vi "IIC Write Bytes.vi"(5 "TimeOutMs":i32, 6 "WriteLen":i32, 7 "pWriteData":u8[](array[numeric])=array[4097 elements], 9 "SlaveAddr":i16, 10 "IICIndex":i32, 11 "DevHandle":i32) -> (2 "function return":i32, 3 "pWriteData out":u8[](array[numeric]))   [LabVIEW 2010, in "usb2iic.lvlib"]
doc: "int WINAPI IIC_WriteBytes(int DevHandle,int IICIndex,short SlaveAddr,unsigned char *pWriteData,int WriteLen,int TimeOutMs);"
uses:
  usb2iic.lvlib
  USB2XXX.dll
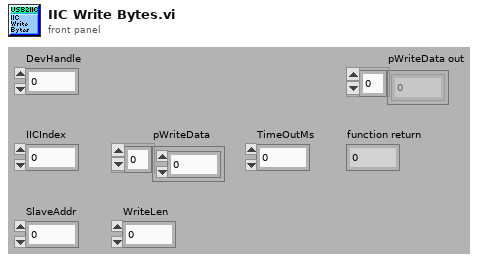
[diagram p1: front panel]
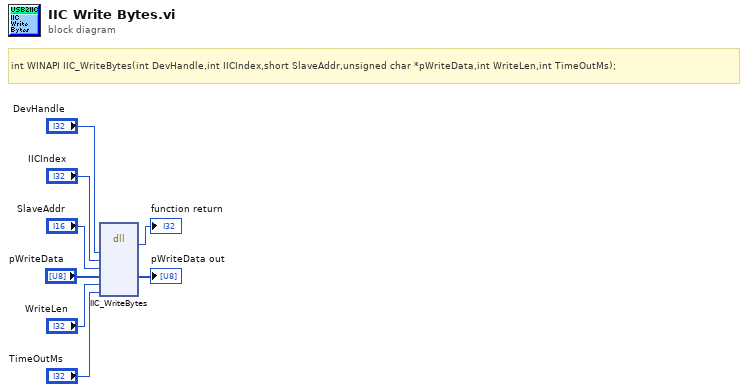
[diagram p0: block diagram]
diagram:
  # "int WINAPI IIC_WriteBytes(int DevHandle,int IICIndex,short SlaveAddr,unsigned char *pWriteData,int WriteLen,int TimeOutMs);"
  n1 = dll-call lib="G:/OtherWork/USB2XXX_Example/trunk/Labview/PublicFiles/USB2XXX.*" fn="IIC_WriteBytes"("DevHandle"="DevHandle", "IICIndex"="IICIndex", "SlaveAddr"="SlaveAddr", "pWriteData"="pWriteData", "WriteLen"="WriteLen", "TimeOutMs"="TimeOutMs") -> (→"function return":i32, "pWriteData"=→"pWriteData out":u8[])  [unwired: 8 in, 2 out]
